vi "Read CB Under Voltage.vi"(8 "error in (no error)":errorcluster, 11 "DC Brick in":refnum<class "DC Brick.lvclass">) -> (0 "error out":errorcluster, 2 "CB Under Voltage":refnum<user-event>, 3 "DC Brick out":refnum<class "DC Brick.lvclass">)   [LabVIEW 2011, in "Tinkerforge.lvlib" / "DC Brick.lvclass"]
uses:
  DC Brick.lvclass
  DC Brick.lvclass/DC Brick.ctl
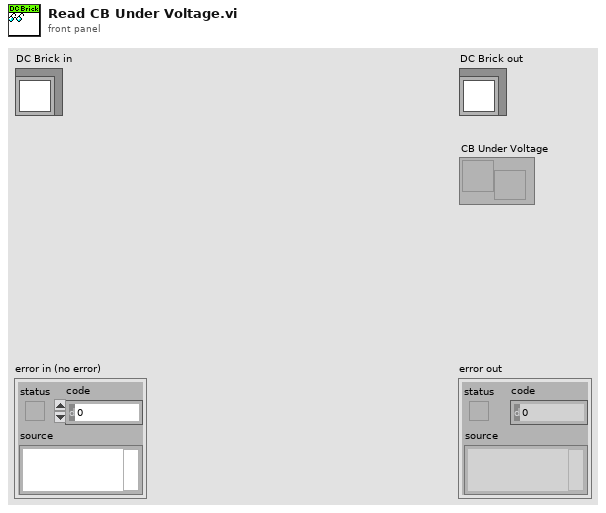
[diagram p1: front panel]
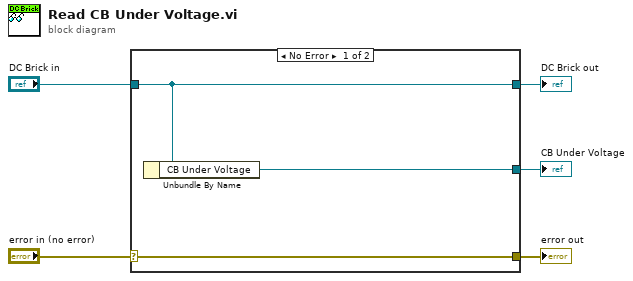
[diagram p0: block diagram]
diagram:
  n1 = case shown="No Error" "error in (no error)" {
    selector: "error in (no error)" -> [w8 w9]
    tunnel: [w8 w9] -> w4
    tunnel: [w7 w10] -> w2
    tunnel: "DC Brick in" -> [w7 w10]
    tunnel: [w6 _] -> w1
    frame No Error {
      n2 = Unbundle By Name(w7) -> ("CB Under Voltage"=w6:refnum<user-event>)
    }
    frame Error {
    }
  }
  "error out" <- w4
  "DC Brick out" <- w2
  "CB Under Voltage" <- w1
